vi "CreateRecord.vi"(6 "Pass_Through_Time":dbl=-1.0 format="%-33.4f", 9 "payload data (little endian)":u8[](array[numeric]), 11 "entry ID":i32) -> (3 "record":u8[](array[numeric]) format="%x")   [LabVIEW 2023]
uses:
  <vilib>/Rock Robotics/WPI/ThirdParty/JAS_Junk/TrajLib/VI/Util_GetTime_U32.vi
  <vilib>/Rock Robotics/WPI/ThirdParty/JAS_Junk/TrajLib/VI/Util_GetTime_U64.vi
  <vilib>/Rock Robotics/WPI/ThirdParty/JAS_Junk/TrajLib/Trajectory_Library.lvlib
panel:
  out "1-byte header length bitfield":u8 format="%0b"
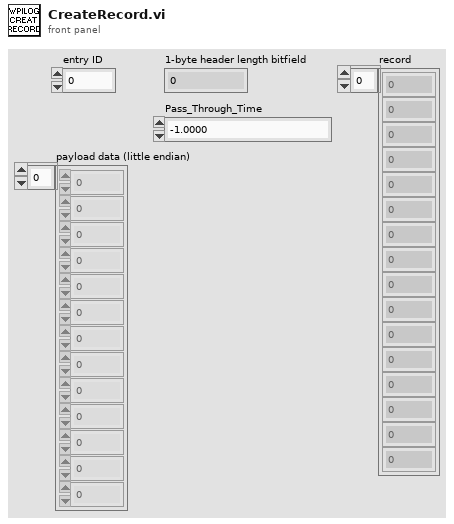
[diagram p1: front panel]
types:
  T1 = enum16{"big-endian, network order", "native, host order", "little-endian"}
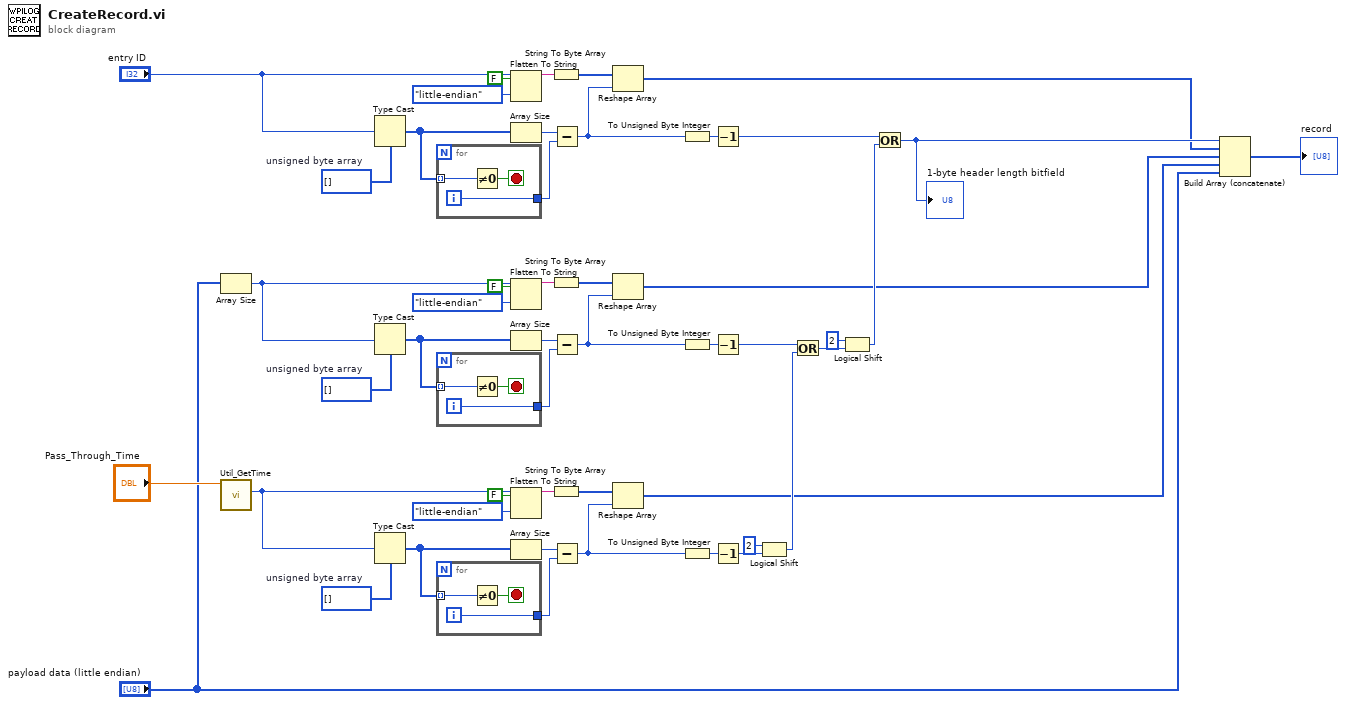
[diagram p0: block diagram]
diagram:
  w11 = u8[] []  # unsigned byte array
  w16 = u8[] []  # unsigned byte array
  w47 = u8[] []  # unsigned byte array
  n1 = Array Size(array="payload data (little endian)") -> (size(s)=w13:i32)
  n2 = call <vilib>:"Util_GetTime.vi"("Pass_Through_Time"="Pass_Through_Time") -> ("FPGA_Time_MicroSeconds"=w32:u64)  [unwired: 8 in, 2 out]
  n3 = Type Cast(type=w11, x="entry ID") -> (*(type *) &x=w9:u8[])
  n4 = Type Cast(type=w16, x=w13) -> (*(type *) &x=w18:u8[])
  n5 = Type Cast(type=w47, x=w32) -> (*(type *) &x=w31:u8[])
  n6 = for {
    tunnel: w9 -> [w51] mode=indexing
    tunnel: [w50] -> w7
    i -> [w50]
    stop <- w49 stop-if-true
    n7 = Not Equal To 0?(x=w51) -> (x != 0?=w49:bool)
  }
  n8 = for {
    tunnel: w18 -> [w54] mode=indexing
    tunnel: [w53] -> w20
    i -> [w53]
    stop <- w52 stop-if-true
    n9 = Not Equal To 0?(x=w54) -> (x != 0?=w52:bool)
  }
  n10 = for {
    tunnel: w31 -> [w57] mode=indexing
    tunnel: [w56] -> w29
    i -> [w56]
    stop <- w55 stop-if-true
    n11 = Not Equal To 0?(x=w57) -> (x != 0?=w55:bool)
  }
  n12 = Flatten To String(anything="entry ID", prepend array or string size? (T)=FALSE, byte order (0:big-endian, network order)=T1."little-endian") -> (data string=w6:string)  [unwired: 1 in, 2 out]
  n13 = Array Size(array=w9) -> (size(s)=w8:i32)
  n14 = Flatten To String(anything=w13, prepend array or string size? (T)=FALSE, byte order (0:big-endian, network order)=T1."little-endian") -> (data string=w21:string)  [unwired: 1 in, 2 out]
  n15 = Array Size(array=w18) -> (size(s)=w19:i32)
  n16 = Flatten To String(anything=w32, prepend array or string size? (T)=FALSE, byte order (0:big-endian, network order)=T1."little-endian") -> (data string=w28:string)  [unwired: 1 in, 2 out]
  n17 = Array Size(array=w31) -> (size(s)=w30:i32)
  n18 = String To Byte Array(string=w6) -> (unsigned byte array=w5:u8[])
  n19 = String To Byte Array(string=w21) -> (unsigned byte array=w22:u8[])
  n20 = String To Byte Array(string=w28) -> (unsigned byte array=w27:u8[])
  n21 = Subtract(x=w8, y=w7) -> (x-y=w2:i32)
  n22 = Subtract(x=w19, y=w20) -> (x-y=w14:i32)
  n23 = Subtract(x=w30, y=w29) -> (x-y=w26:i32)
  n24 = Reshape Array(w5, w2) -> (w1:u8[])
  n25 = Reshape Array(w22, w14) -> (w15:u8[])
  n26 = Reshape Array(w27, w26) -> (w25:u8[])
  n27 = To Unsigned Byte Integer(number=w2) -> (unsigned 8bit integer=w37:u8)
  n28 = To Unsigned Byte Integer(number=w14) -> (unsigned 8bit integer=w36:u8)
  n29 = To Unsigned Byte Integer(number=w26) -> (unsigned 8bit integer=w35:u8)
  n30 = Decrement(x=w37) -> (x-1=w41:u8)
  n31 = Decrement(x=w36) -> (x-1=w44:u8)
  n32 = Decrement(x=w35) -> (x-1=w39:u8)
  n33 = Logical Shift(y=i16 2, x=w39) -> (x << y=w45:u8)
  n34 = Or(x=w44, y=w45) -> (x .or. y?=w42:u8)
  n35 = Logical Shift(y=i16 2, x=w42) -> (x << y=w40:u8)
  n36 = Or(x=w41, y=w40) -> (x .or. y?=w38:u8)
  "1-byte header length bitfield" <- w38
  n37 = Build Array (concatenate)(w38, w1, w15, w25, "payload data (little endian)") -> (→"record":u8[])
